vi "Formula.vi"() -> ()   [LabVIEW 2023]
panel:
  out "outputVariable":dbl
  out "x+y":dbl
  in  "Numeric2":dbl
  in  "Numeric":dbl
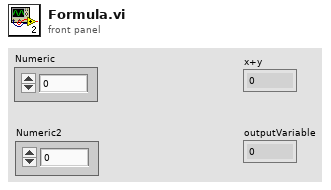
[diagram p1: front panel]
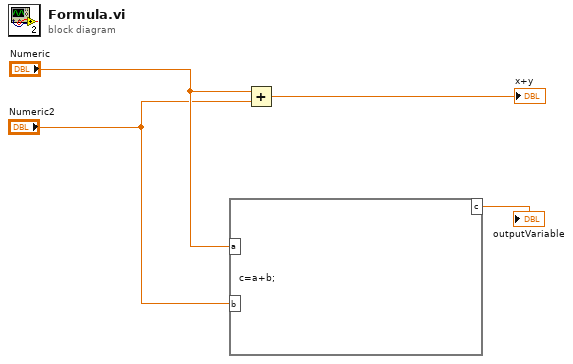
[diagram p0: block diagram]
diagram:
  n1 = formula code="c=a+b;"("a"="Numeric", "b"="Numeric2") -> ("c"=→"outputVariable":dbl)
  n2 = Add(x="Numeric", y="Numeric2") -> (x+y=→"x+y":dbl)
